vi "picoscopeUpdateSettings.vi"(8 "error in (no error)":errorcluster, 11 "PicoscopeV2 in":refnum<class "PicoscopeV2.lvclass">) -> (0 "error out":errorcluster, 3 "PicoscopeV2 out":refnum<class "PicoscopeV2.lvclass">)   [LabVIEW 2020, in "PicoscopeV2.lvclass"]
uses:
  PicoscopeV2.lvclass
  PicoscopeV2.lvclass/PicoscopeV2.ctl
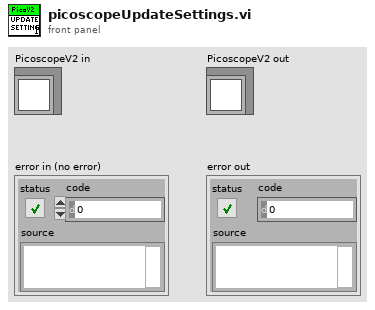
[diagram p1: front panel]
types:
  T1 = typedef "PicoScope5000aDigitalChannelSettings.ctl" = cluster{"Enabled":bool, "Logic Level":i16}
  T2 = typedef "PicoScope5000aAnalogChannelSettings.ctl" = cluster{"Enabled":bool, "Coupling":i16, "Range":u16, "Analogue Offset":sgl, "Bandwidth Limit":u32}
  T3 = cluster{"Trigger Enabled":bool, "Trigger Source":enum16{"Channel A", "Channel B", "Channel C", "Channel D", "Ext."}, "Trigger Threshold (volts)":dbl, "Trigger Direction":u16, "Trigger Delay (samples)":u32, "Auto Trigger Time (ms)":i16}
  T4 = cluster{"Driver Version":string, "USB Version":string, "Hardware":string, "Variant":string, "Batch and Serial":string, "Cal Date":string, "Kernel Version":string, "Digital HW Version":string, "Analogue HW Version":string, "MSO":bool, "Number of channels":i16}
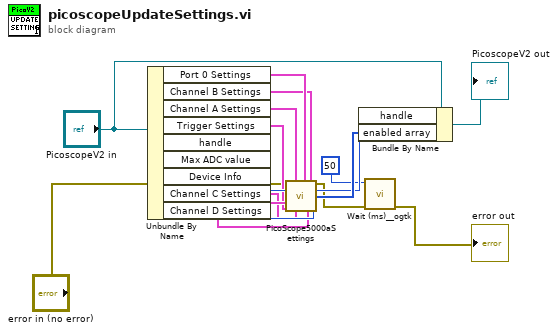
[diagram p0: block diagram]
diagram:
  n1 = Unbundle By Name("PicoscopeV2 in") -> ("Port 0 Settings"=w13:T1, "Channel B Settings"=w12:T2, "Channel A Settings"=w11:T2, "Trigger Settings"=w5:T3, "handle"=w8:i16, "Max ADC value"=w9:i16, "Device Info"=w10:T4, "Channel C Settings"=w2:T2, "Channel D Settings"=w1:T2)
  n2 = call "PicoScope5000aSettings.vi"("error in"="error in (no error)", "Channel A Settings"=w11, "Port 0 Settings"=w13, "Channel B Settings"=w12, "handle in"=w8, "Device Info"=w10, "Trigger Settings"=w5, "Channel C Settings"=w2, "Channel D Settings"=w1, "Max ADC value"=w9) -> ("error out"=w6:errorcluster, "handle out"=w15:i16, "enabled array"=w16:i16[])  [unwired: 3 in]
  n3 = Bundle By Name(cluster="PicoscopeV2 in", "handle"=w15, "enabled array"=w16) -> (→"PicoscopeV2 out":refnum<class "PicoscopeV2.lvclass">)
  n4 = call "Wait (ms)__ogtk.vi"("error in (no error)"=w6, "milliseconds to wait"=u32 50) -> ("error out"=→"error out":errorcluster)  [unwired: 8 in, 1 out]
